vi "Sequential.vi"   [LabVIEW 2011]
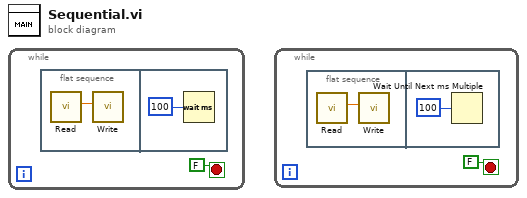
[diagram p0: block diagram]
diagram:
  n1 = while {
    stop <- FALSE stop-if-true
    n2 = flat-sequence {
      frame #0 {
        n3 = call "Read.vi"() -> ("Numeric"=w2:dbl)  [unwired: 11 in]
        n4 = call "Write.vi"("Numeric"=w2) -> ()  [unwired: 11 in]
      }
      frame #1 {
        n5 = Wait (ms)(milliseconds to wait=u32 100) -> ()  [unwired: 1 out]
      }
    }
  }
  n6 = while {
    stop <- FALSE stop-if-true
    n7 = flat-sequence {
      frame #0 {
        n8 = call "Read.vi"() -> ("Numeric"=w5:dbl)  [unwired: 11 in]
        n9 = call "Write.vi"("Numeric"=w5) -> ()  [unwired: 11 in]
      }
      frame #1 {
        n10 = Wait Until Next ms Multiple(millisecond multiple=u32 100) -> ()  [unwired: 1 out]
      }
    }
  }
